vi "Autonomous Independent V.3.0.vi"() -> ()   [LabVIEW 2017]
doc: "This VI is called when autonomous begins, and will automatically be terminated when autonomous ends. You can carry out timed or sensor driven robot movement independently without needing to return to the caller."
uses:
  <vilib>/Rock Robotics/Network Tables/NT Read String.vi
  Robot Global Data V.3.0.vi
panel:
  out "Collector and Drive Loop Run Speed":dbl
  # "Be sure to right-click and choose Data Operations>>Make Current Value default if you want to save the array values with the VI"
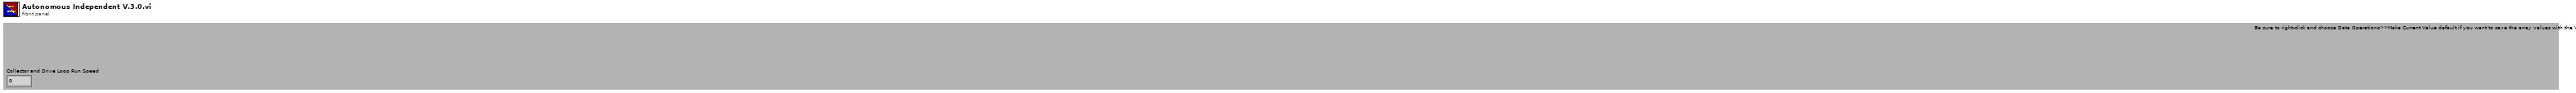
[diagram p1: front panel]
types:
  T1 = typedef "WPI_GyroDevRef.ctl" = cluster{"DevStatus":errorcluster, "Analog Channel":T2, "Gain (VoltsPerDegree/Second)":dbl, "Gyro Type":enum16{"Analog", "XRS450"}, "Handle":i32, "SPI Bus":T3, "Device Found":bool, "Sample Rate":dbl, "Calibrate On Open":bool, "Offset":dbl}
  T2 = typedef "FPGA_AIChannel.ctl" = enum8{"AI 0", "AI 1", "AI 2", "AI 3", "AI MXP 0", "AI MXP 1", "AI MXP 2", "AI MXP 3", "Invalid"}
  T3 = typedef "spi_bus.ctl" = enum16{"SPI On-Board, CS0", "SPI On-Board, CS1", "SPI On-Board, CS2", "SPI On-Board, CS3", "SPI MXP", "Invalid"}
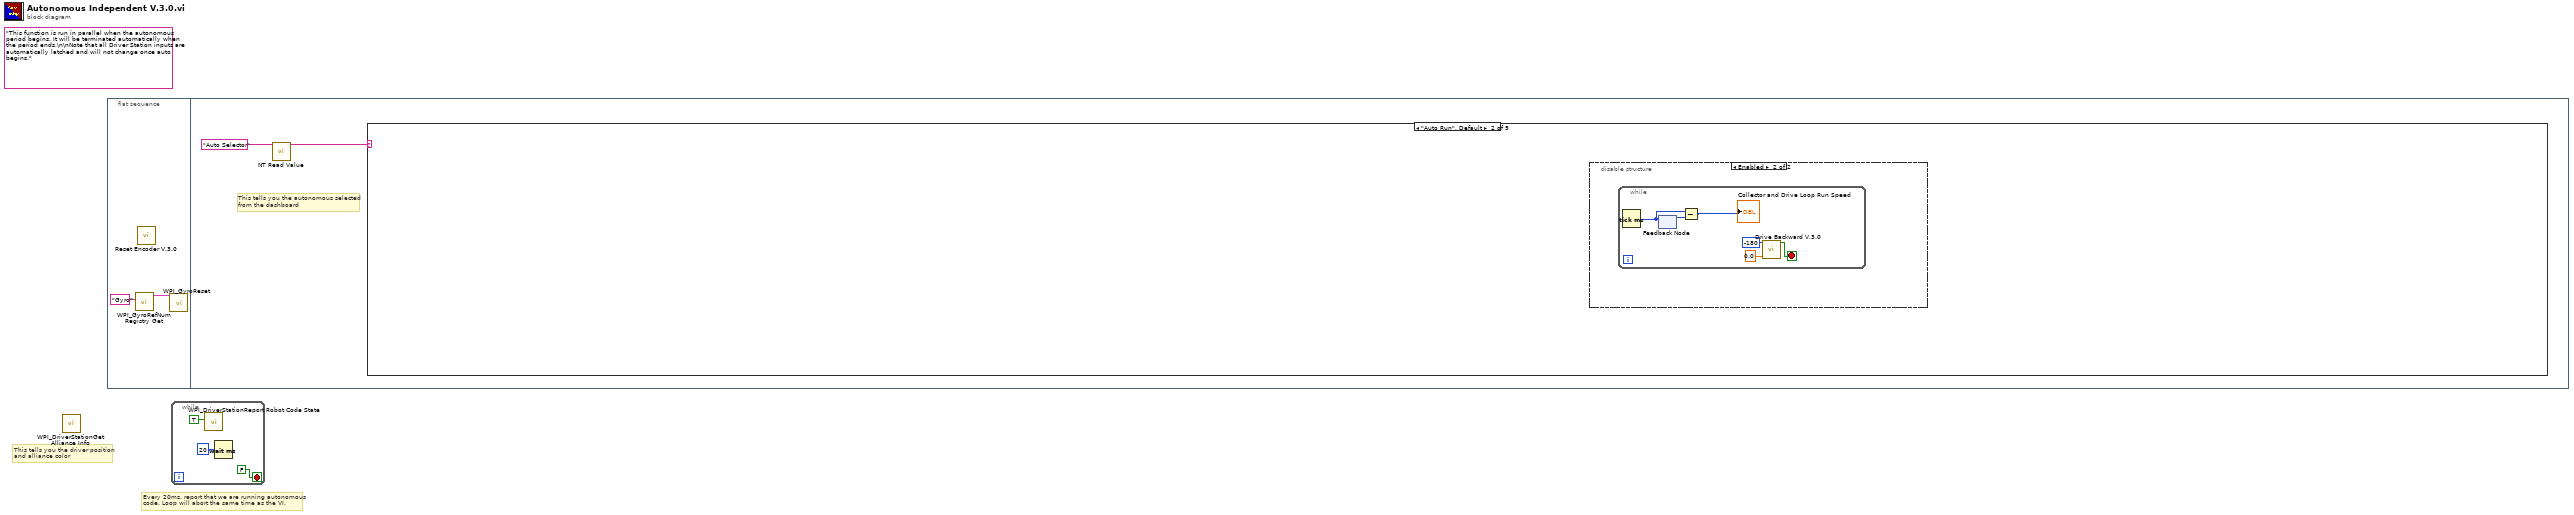
[diagram p0: block diagram]
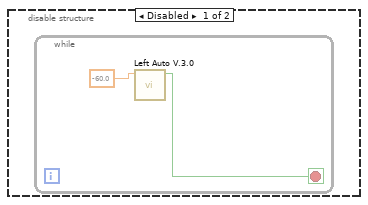
[diagram p3: hidden frame]
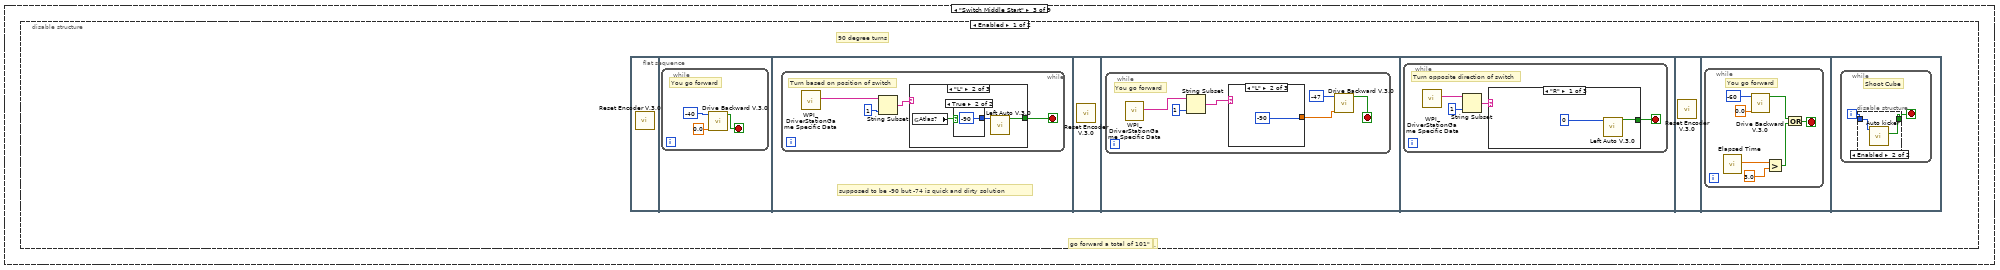
[diagram p4: hidden frame]
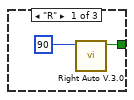
[diagram p5: hidden frame]
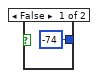
[diagram p6: hidden frame]
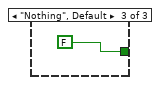
[diagram p7: hidden frame]
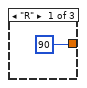
[diagram p8: hidden frame]
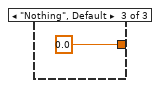
[diagram p9: hidden frame]
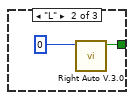
[diagram p10: hidden frame]
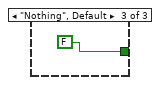
[diagram p11: hidden frame]
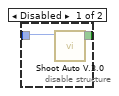
[diagram p12: hidden frame]
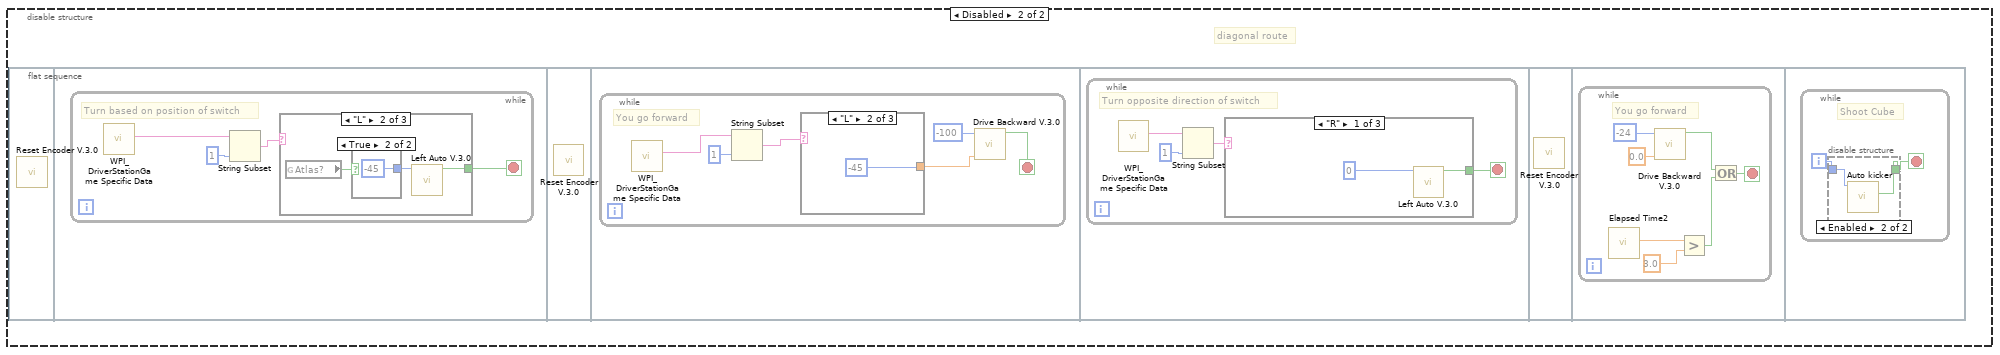
[diagram p13: hidden frame]
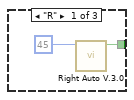
[diagram p14: hidden frame]
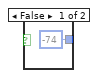
[diagram p15: hidden frame]
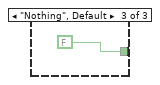
[diagram p16: hidden frame]
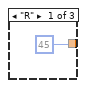
[diagram p17: hidden frame]
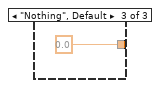
[diagram p18: hidden frame]
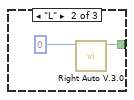
[diagram p19: hidden frame]
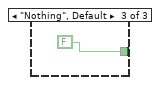
[diagram p20: hidden frame]
diagram:
  (unwired) "This function is run in parallel when the autonomous period begins. It will be terminated automatically when the period ends.\n\nNote that all Driver Station inputs are automatically latched and will not change once auto begins."
  # "This tells you the driver position\nand alliance color"
  # "Every 20ms, report that we are running autonomous\ncode. Loop will abort the same time as the VI."
  n1 = call <vilib>:"WPI_DriverStationGet Alliance Info.vi"() -> ()  [unwired: 12 out]
  n2 = flat-sequence {
    frame #0 {
      n3 = call <vilib>:"WPI_GyroRefNum Registry Get.vi"("refnum name"="Gyro") -> ("GyroDevRef"=w2:T1)  [unwired: 9 in, 1 out]
      n4 = call "Reset Encoder V.3.0.vi"() -> ()  [unwired: 12 in]
      n5 = call <vilib>:"WPI_GyroReset.vi"("GyroDevRef"=w2) -> ()  [unwired: 9 in, 2 out]
    }
    frame #1 {
      # "This tells you the autonomous selected\nfrom the dashboard"
      n6 = call-poly <vilib>:"NT Read Value.vi"("Name"="Auto Selector") -> ("String"=w3:string)  [unwired: 9 in, 1 out]
      n7 = case shown="\"Auto Run\", Default" w3 {
        frame "Nothing" {
          # "You can put your main auto here, or you can right-click on the case and make any\nother frame be the default case."
          # "This is the frame that will execute if no selection is made, or if it is not recognized"
        }
        frame "Auto Run", Default {
          n8 = disable-structure shown="Enabled" {
            frame Disabled {
              n9 = while {
                stop <- w5 stop-if-true
                n10 = call "Left Auto V.3.0.vi"("Desired Angle"=-60.0) -> ("Stop"=w5:bool)  [unwired: 10 in]
              }
            }
            frame Enabled {
              n11 = while {
                stop <- w11 stop-if-true
                n12 = Tick Count (ms)() -> (millisecond timer value=w9:u32)
                n13 = feedback #1() -> (w10:u32)  [unwired: 1 in]
                n14 = feedback-in #1(w9) -> ()
                n15 = Subtract(x=w9, y=w10) -> (x-y=→"Collector and Drive Loop Run Speed":u32)
                n16 = call "Drive Backward V.3.0.vi"("Desired Angle"=0.0, "Encoder Distance (in.)"=-180) -> ("Stop"=w11:bool)  [unwired: 9 in]
              }
            }
          }
        }
        frame "Switch Middle Start" {
          n17 = disable-structure shown="Enabled" {
            frame Enabled {
              # "90 degree turns"
              # "."
              # "go forward a total of 101\""
              n18 = flat-sequence {
                frame #0 {
                  n19 = call "Reset Encoder V.3.0.vi"() -> ()  [unwired: 12 in]
                }
                frame #1 {
                  n20 = while {
                    stop <- w14 stop-if-true
                    # "You go forward"
                    n21 = call "Drive Backward V.3.0.vi"("Desired Angle"=0.0, "Encoder Distance (in.)"=-40) -> ("Stop"=w14:bool)  [unwired: 9 in]
                  }
                }
                frame #2 {
                  # "supposed to be -90 but -74 is quick and dirty solution"
                  n22 = while {
                    stop <- w16 stop-if-true
                    # "Turn based on position of switch"
                    n23 = call <vilib>:"WPI_DriverStationGame Specific Data.vi"() -> ("Game Specific Data"=w19:string)  [unwired: 11 in]
                    n24 = String Subset(string=w19, length (rest)=1 ("length (rest)")) -> (substring=w17:string)  [unwired: 1 in]
                    n25 = case shown="\"L\"" w17 {
                      tunnel: [w20 w23 FALSE] -> w16
                      frame "R" {
                        n26 = call "Right Auto V.3.0.vi"("Desired Angle"=90) -> ("Stop"=w20:bool)  [unwired: 9 in]
                      }
                      frame "L" {
                        n27 = global read "Robot Global Data V.3.0.vi" "Atlas?"() -> (w22:bool)
                        n28 = case shown="True" w22 {
                          tunnel: [-74 -90] -> w24
                          frame False {
                          }
                          frame True {
                          }
                        }
                        n29 = call "Left Auto V.3.0.vi"("Desired Angle"=w24) -> ("Stop"=w23:bool)  [unwired: 10 in]
                      }
                      frame "Nothing", Default {
                      }
                    }
                  }
                }
                frame #3 {
                  n30 = call "Reset Encoder V.3.0.vi"() -> ()  [unwired: 12 in]
                }
                frame #4 {
                  n31 = while {
                    stop <- w32 stop-if-true
                    # "You go forward"
                    n32 = call <vilib>:"WPI_DriverStationGame Specific Data.vi"() -> ("Game Specific Data"=w30:string)  [unwired: 11 in]
                    n33 = String Subset(string=w30, length (rest)=1 ("length (rest)")) -> (substring=w31:string)  [unwired: 1 in]
                    n34 = case shown="\"L\"" w31 {
                      tunnel: [90 -90 0.0] -> w28
                      frame "R" {
                      }
                      frame "L" {
                      }
                      frame "Nothing", Default {
                      }
                    }
                    n35 = call "Drive Backward V.3.0.vi"("Desired Angle"=w28, "Encoder Distance (in.)"=-47) -> ("Stop"=w32:bool)  [unwired: 9 in]
                  }
                }
                frame #5 {
                  n36 = while {
                    stop <- w37 stop-if-true
                    # "Turn opposite direction of switch"
                    n37 = call <vilib>:"WPI_DriverStationGame Specific Data.vi"() -> ("Game Specific Data"=w40:string)  [unwired: 11 in]
                    n38 = String Subset(string=w40, length (rest)=1 ("length (rest)")) -> (substring=w38:string)  [unwired: 1 in]
                    n39 = case shown="\"R\"" w38 {
                      tunnel: [w41 w43 FALSE] -> w37
                      frame "R" {
                        n40 = call "Left Auto V.3.0.vi"("Desired Angle"=0) -> ("Stop"=w41:bool)  [unwired: 10 in]
                      }
                      frame "L" {
                        n41 = call "Right Auto V.3.0.vi"("Desired Angle"=0) -> ("Stop"=w43:bool)  [unwired: 9 in]
                      }
                      frame "Nothing", Default {
                      }
                    }
                  }
                }
                frame #6 {
                  n42 = call "Reset Encoder V.3.0.vi"() -> ()  [unwired: 12 in]
                }
                frame #7 {
                  n43 = while {
                    stop <- w50 stop-if-true
                    # "You go forward"
                    n44 = call "Elapsed Time"() -> ("Elapsed Time (s)"=w48:dbl)  [unwired: 12 in, 7 out]
                    n45 = call "Drive Backward V.3.0.vi"("Desired Angle"=0.0, "Encoder Distance (in.)"=-60) -> ("Stop"=w46:bool)  [unwired: 9 in]
                    n46 = Greater?(x=w48, y=3.0) -> (0:w47:bool)
                    n47 = Or(x=w46, y=w47) -> (x .or. y?=w50:bool)
                  }
                }
                frame #8 {
                  n48 = while {
                    i -> [w54]
                    stop <- w53 stop-if-true
                    # "Shoot Cube"
                    n49 = disable-structure shown="Enabled" {
                      disable-tunnel: w54 -> [w56 w58]
                      disable-tunnel: [w55 w57] -> w53
                      frame Disabled {
                        n50 = call "Shoot Auto V.3.0.vi"("Iteration"=w56) -> ("Stop"=w55:bool)  [unwired: 10 in]
                      }
                      frame Enabled {
                        n51 = call "Auto kicker.vi"("Iteration"=w58) -> ("Stop"=w57:bool)  [unwired: 10 in]
                      }
                    }
                  }
                }
              }
            }
            frame Disabled {
              # "diagonal route"
              n52 = flat-sequence {
                frame #0 {
                  n53 = call "Reset Encoder V.3.0.vi"() -> ()  [unwired: 12 in]
                }
                frame #1 {
                  n54 = while {
                    stop <- w59 stop-if-true
                    # "Turn based on position of switch"
                    n55 = call <vilib>:"WPI_DriverStationGame Specific Data.vi"() -> ("Game Specific Data"=w62:string)  [unwired: 11 in]
                    n56 = String Subset(string=w62, length (rest)=1 ("length (rest)")) -> (substring=w60:string)  [unwired: 1 in]
                    n57 = case shown="\"L\"" w60 {
                      tunnel: [w63 w66 FALSE] -> w59
                      frame "R" {
                        n58 = call "Right Auto V.3.0.vi"("Desired Angle"=45) -> ("Stop"=w63:bool)  [unwired: 9 in]
                      }
                      frame "L" {
                        n59 = global read "Robot Global Data V.3.0.vi" "Atlas?"() -> (w65:bool)
                        n60 = case shown="True" w65 {
                          tunnel: [-74 -45] -> w67
                          frame False {
                          }
                          frame True {
                          }
                        }
                        n61 = call "Left Auto V.3.0.vi"("Desired Angle"=w67) -> ("Stop"=w66:bool)  [unwired: 10 in]
                      }
                      frame "Nothing", Default {
                      }
                    }
                  }
                }
                frame #2 {
                  n62 = call "Reset Encoder V.3.0.vi"() -> ()  [unwired: 12 in]
                }
                frame #3 {
                  n63 = while {
                    stop <- w75 stop-if-true
                    # "You go forward"
                    n64 = call <vilib>:"WPI_DriverStationGame Specific Data.vi"() -> ("Game Specific Data"=w73:string)  [unwired: 11 in]
                    n65 = String Subset(string=w73, length (rest)=1 ("length (rest)")) -> (substring=w74:string)  [unwired: 1 in]
                    n66 = case shown="\"L\"" w74 {
                      tunnel: [45 -45 0.0] -> w71
                      frame "R" {
                      }
                      frame "L" {
                      }
                      frame "Nothing", Default {
                      }
                    }
                    n67 = call "Drive Backward V.3.0.vi"("Desired Angle"=w71, "Encoder Distance (in.)"=-100) -> ("Stop"=w75:bool)  [unwired: 9 in]
                  }
                }
                frame #4 {
                  n68 = while {
                    stop <- w80 stop-if-true
                    # "Turn opposite direction of switch"
                    n69 = call <vilib>:"WPI_DriverStationGame Specific Data.vi"() -> ("Game Specific Data"=w83:string)  [unwired: 11 in]
                    n70 = String Subset(string=w83, length (rest)=1 ("length (rest)")) -> (substring=w81:string)  [unwired: 1 in]
                    n71 = case shown="\"R\"" w81 {
                      tunnel: [w84 w86 FALSE] -> w80
                      frame "R" {
                        n72 = call "Left Auto V.3.0.vi"("Desired Angle"=0) -> ("Stop"=w84:bool)  [unwired: 10 in]
                      }
                      frame "L" {
                        n73 = call "Right Auto V.3.0.vi"("Desired Angle"=0) -> ("Stop"=w86:bool)  [unwired: 9 in]
                      }
                      frame "Nothing", Default {
                      }
                    }
                  }
                }
                frame #5 {
                  n74 = call "Reset Encoder V.3.0.vi"() -> ()  [unwired: 12 in]
                }
                frame #6 {
                  n75 = while {
                    stop <- w93 stop-if-true
                    # "You go forward"
                    n76 = call "Elapsed Time2"() -> ("Elapsed Time (s)"=w91:dbl)  [unwired: 12 in, 7 out]
                    n77 = call "Drive Backward V.3.0.vi"("Desired Angle"=0.0, "Encoder Distance (in.)"=-24) -> ("Stop"=w89:bool)  [unwired: 9 in]
                    n78 = Greater?(x=w91, y=3.0) -> (0:w90:bool)
                    n79 = Or(x=w89, y=w90) -> (x .or. y?=w93:bool)
                  }
                }
                frame #7 {
                  n80 = while {
                    i -> [w97]
                    stop <- w96 stop-if-true
                    # "Shoot Cube"
                    n81 = disable-structure shown="Enabled" {
                      disable-tunnel: w97 -> [w99 w101]
                      disable-tunnel: [w98 w100] -> w96
                      frame Disabled {
                        n82 = call "Shoot Auto V.3.0.vi"("Iteration"=w99) -> ("Stop"=w98:bool)  [unwired: 10 in]
                      }
                      frame Enabled {
                        n83 = call "Auto kicker.vi"("Iteration"=w101) -> ("Stop"=w100:bool)  [unwired: 10 in]
                      }
                    }
                  }
                }
              }
            }
          }
        }
        frame "Switch Optimize Left Start" {
          # "Read Switch Side"
          n84 = call <vilib>:"WPI_DriverStationGame Specific Data.vi"() -> ("Game Specific Data"=w104:string)  [unwired: 11 in]
          n85 = String Subset(string=w104, length (rest)=1 ("length (rest)")) -> (substring=w102:string)  [unwired: 1 in]
          n86 = case shown="\"R\"" w102 {
            frame "Nothing", Default {
            }
            frame "R" {
              w106 = 1 ("length (rest)")
              # "switch on other side, check scale"
              n87 = call <vilib>:"WPI_DriverStationGame Specific Data.vi"() -> ("Game Specific Data"=w107:string)  [unwired: 11 in]
              n88 = String Subset(string=w107, offset (0)=w106, length (rest)=w106) -> (substring=w105:string)
              n89 = case shown="\"L\"" w105 {
                frame "Nothing", Default {
                }
                frame "L" {
                  # "Scale on our side, do it"
                  n90 = flat-sequence {
                    frame #0 {
                      n91 = call "Reset Encoder V.3.0.vi"() -> ()  [unwired: 12 in]
                    }
                    frame #1 {
                      n92 = while {
                        stop <- w109 stop-if-true
                        # "You go forward"
                        n93 = call "Drive Backward V.3.0.vi"("Desired Angle"=0.0, "Encoder Distance (in.)"=-262) -> ("Stop"=w109:bool)  [unwired: 9 in]
                      }
                    }
                    frame #2 {
                      n94 = flat-sequence {
                        frame #0 {
                          n95 = while {
                            stop <- w113 stop-if-true
                            # "Turn right slightly"
                            n96 = call "Right Auto V.3.0.vi"("Desired Angle"=60) -> ("Stop"=w113:bool)  [unwired: 9 in]
                          }
                        }
                        frame #1 {
                          n97 = call "Reset Encoder V.3.0.vi"() -> ()  [unwired: 12 in]
                        }
                        frame #2 {
                          n98 = while {
                            stop <- w116 stop-if-true
                            # "Forward"
                            n99 = call "Drive Backward V.3.0.vi"("Desired Angle"=60.0, "Encoder Distance (in.)"=-16) -> ("Stop"=w116:bool)  [unwired: 9 in]
                          }
                        }
                      }
                      n100 = while {
                        stop <- w111 stop-if-true
                        # "Raise Darts"
                        n101 = call "Dart Auto V.3.0.vi"() -> ("Stop"=w111:bool)  [unwired: 11 in]
                      }
                    }
                    frame #3 {
                      n102 = call "Reset Encoder V.3.0.vi"() -> ()  [unwired: 12 in]
                    }
                    frame #4 {
                      n103 = disable-structure shown="Enabled" {
                        frame Enabled {
                          n104 = while {
                            stop <- w121 stop-if-true
                            # "Move Backward"
                            n105 = call "Forward Auto V.3.0.vi"("Desired Angle"=90.0, "Encoder Distance (in.)"=30.0 ("Encoder Distance")) -> ("Stop"=w121:bool)  [unwired: 9 in]
                          }
                          n106 = flat-sequence {
                            frame #0 {
                              n107 = while {
                                i -> [w118]
                                stop <- w117 stop-if-true
                                # "Shoot Cube"
                                n108 = call "Shoot Auto V.3.0.vi"("Iteration"=w118) -> ("Stop"=w117:bool)  [unwired: 10 in]
                              }
                            }
                            frame #1 {
                              n109 = while {
                                stop <- w119 stop-if-true
                                n110 = call "Auto Arms Down V.3.0.vi"() -> ("Stop"=w119:bool)  [unwired: 11 in]
                              }
                            }
                          }
                        }
                        frame Disabled {
                        }
                      }
                    }
                    frame #5 {
                      n111 = disable-structure shown="Disabled" {
                        frame Disabled {
                          n112 = while {
                            stop <- w124 stop-if-true
                            # "Turn right slightly"
                            n113 = call "Right Auto V.3.0.vi"("Desired Angle"=-30) -> ("Stop"=w124:bool)  [unwired: 9 in]
                          }
                        }
                        frame Enabled {
                        }
                      }
                    }
                  }
                }
                frame "R" {
                  # "Scale on other side, do it anyway"
                  n114 = flat-sequence {
                    frame #0 {
                      n115 = call "Reset Encoder V.3.0.vi"() -> ()  [unwired: 12 in]
                    }
                    frame #1 {
                      n116 = while {
                        stop <- w126 stop-if-true
                        # "Forward"
                        n117 = call "Drive Backward V.3.0.vi"("Desired Angle"=0.0, "Encoder Distance (in.)"=-232) -> ("Stop"=w126:bool)  [unwired: 9 in]
                      }
                    }
                    frame #2 {
                      n118 = while {
                        stop <- w129 stop-if-true
                        # "Right"
                        n119 = call "Right Auto V.3.0.vi"("Desired Angle"=90) -> ("Stop"=w129:bool)  [unwired: 9 in]
                      }
                    }
                    frame #3 {
                      n120 = call "Reset Encoder V.3.0.vi"() -> ()  [unwired: 12 in]
                    }
                    frame #4 {
                      n121 = while {
                        stop <- w131 stop-if-true
                        # "Forward"
                        n122 = call "Drive Backward V.3.0.vi"("Desired Angle"=90.0, "Encoder Distance (in.)"=-200) -> ("Stop"=w131:bool)  [unwired: 9 in]
                      }
                    }
                    frame #5 {
                      n123 = flat-sequence {
                        frame #0 {
                          n124 = while {
                            stop <- w135 stop-if-true
                            # "Left"
                            n125 = call "Left Auto V.3.0.vi"("Desired Angle"=0) -> ("Stop"=w135:bool)  [unwired: 10 in]
                          }
                        }
                        frame #1 {
                          n126 = call "Reset Encoder V.3.0.vi"() -> ()  [unwired: 12 in]
                        }
                        frame #2 {
                          n127 = disable-structure shown="Disabled" {
                            frame Disabled {
                              n128 = while {
                                stop <- w138 stop-if-true
                                # "Forward"
                                n129 = call "Drive Backward V.3.0.vi"("Desired Angle"=0.0, "Encoder Distance (in.)"=-49) -> ("Stop"=w138:bool)  [unwired: 9 in]
                              }
                            }
                            frame Enabled {
                            }
                          }
                        }
                      }
                      n130 = while {
                        stop <- w133 stop-if-true
                        # "Raise Darts"
                        n131 = call "Dart Auto V.3.0.vi"() -> ("Stop"=w133:bool)  [unwired: 11 in]
                      }
                    }
                    frame #6 {
                      n132 = disable-structure shown="Disabled" {
                        frame Disabled {
                          n133 = while {
                            i -> [w140]
                            stop <- w139 stop-if-true
                            # "Shoot Cube"
                            n134 = call "Shoot Auto V.3.0.vi"("Iteration"=w140) -> ("Stop"=w139:bool)  [unwired: 10 in]
                          }
                        }
                        frame Enabled {
                        }
                      }
                    }
                    frame #7 {
                      n135 = call "Reset Encoder V.3.0.vi"() -> ()  [unwired: 12 in]
                    }
                    frame #8 {
                      n136 = disable-structure shown="Disabled" {
                        frame Disabled {
                          n137 = while {
                            stop <- w143 stop-if-true
                            # "Move Backward"
                            n138 = call "Forward Auto V.3.0.vi"("Desired Angle"=0.0, "Encoder Distance (in.)"=10.0 ("Encoder Distance")) -> ("Stop"=w143:bool)  [unwired: 9 in]
                          }
                          n139 = while {
                            stop <- w141 stop-if-true
                            n140 = call "Auto Arms Down V.3.0.vi"() -> ("Stop"=w141:bool)  [unwired: 11 in]
                          }
                        }
                        frame Enabled {
                        }
                      }
                    }
                  }
                }
              }
            }
            frame "L" {
              # "Switch on our side, do switch"
              n141 = flat-sequence {
                frame #0 {
                  n142 = call "Reset Encoder V.3.0.vi"() -> ()  [unwired: 12 in]
                }
                frame #1 {
                  n143 = while {
                    stop <- w147 stop-if-true
                    # "was -183"
                    n144 = call "Drive Backward V.3.0.vi"("Desired Angle"=0.0, "Encoder Distance (in.)"=-162.0) -> ("Stop"=w147:bool)  [unwired: 9 in]
                  }
                }
                frame #2 {
                  n145 = while {
                    stop <- w149 stop-if-true
                    n146 = call "Right Auto V.3.0.vi"("Desired Angle"=90.0) -> ("Stop"=w149:bool)  [unwired: 9 in]
                  }
                }
                frame #3 {
                  n147 = call "Reset Encoder V.3.0.vi"() -> ()  [unwired: 12 in]
                }
                frame #4 {
                  n148 = while {
                    stop <- w150 stop-if-true
                    # "was  -16"
                    n149 = call "Drive Backward V.3.0.vi"("Desired Angle"=90.0, "Encoder Distance (in.)"=-22.0) -> ("Stop"=w150:bool)  [unwired: 9 in]
                  }
                }
                frame #5 {
                  n150 = while {
                    i -> [w153]
                    stop <- w154 stop-if-true
                    n151 = call "Shoot Auto V.3.0.vi"("Iteration"=w153) -> ("Stop"=w154:bool)  [unwired: 10 in]
                  }
                }
              }
            }
          }
        }
        frame "Switch Optimize Right Start" {
          # "Read Switch"
          n152 = call <vilib>:"WPI_DriverStationGame Specific Data.vi"() -> ("Game Specific Data"=w157:string)  [unwired: 11 in]
          n153 = String Subset(string=w157, length (rest)=1 ("length (rest)")) -> (substring=w155:string)  [unwired: 1 in]
          n154 = case shown="\"L\"" w155 {
            frame "Nothing", Default {
            }
            frame "R" {
              # "Switch on our side, do it"
              n155 = flat-sequence {
                frame #0 {
                  n156 = call "Reset Encoder V.3.0.vi"() -> ()  [unwired: 12 in]
                }
                frame #1 {
                  n157 = while {
                    stop <- w160 stop-if-true
                    # "was -183"
                    n158 = call "Drive Backward V.3.0.vi"("Desired Angle"=0.0, "Encoder Distance (in.)"=-162.0) -> ("Stop"=w160:bool)  [unwired: 9 in]
                  }
                }
                frame #2 {
                  n159 = while {
                    stop <- w162 stop-if-true
                    n160 = call "Right Auto V.3.0.vi"("Desired Angle"=90.0) -> ("Stop"=w162:bool)  [unwired: 9 in]
                  }
                }
                frame #3 {
                  n161 = call "Reset Encoder V.3.0.vi"() -> ()  [unwired: 12 in]
                }
                frame #4 {
                  n162 = while {
                    stop <- w163 stop-if-true
                    # "was  -16"
                    n163 = call "Drive Backward V.3.0.vi"("Desired Angle"=90.0, "Encoder Distance (in.)"=-22.0) -> ("Stop"=w163:bool)  [unwired: 9 in]
                  }
                }
                frame #5 {
                  n164 = while {
                    i -> [w166]
                    stop <- w167 stop-if-true
                    n165 = call "Shoot Auto V.3.0.vi"("Iteration"=w166) -> ("Stop"=w167:bool)  [unwired: 10 in]
                  }
                }
              }
            }
            frame "L" {
              w169 = 1 ("length (rest)")
              # "Switch on wrong side, read\nscale"
              n166 = call <vilib>:"WPI_DriverStationGame Specific Data.vi"() -> ("Game Specific Data"=w170:string)  [unwired: 11 in]
              n167 = String Subset(string=w170, offset (0)=w169, length (rest)=w169) -> (substring=w168:string)
              n168 = case shown="\"R\"" w168 {
                frame "Nothing", Default {
                }
                frame "R" {
                  # "Scale on same side - do it"
                  n169 = flat-sequence {
                    frame #0 {
                      n170 = call "Reset Encoder V.3.0.vi"() -> ()  [unwired: 12 in]
                    }
                    frame #1 {
                      # "was -277"
                      n171 = while {
                        stop <- w172 stop-if-true
                        # "You go forward"
                        n172 = call "Drive Backward V.3.0.vi"("Desired Angle"=0.0, "Encoder Distance (in.)"=-262) -> ("Stop"=w172:bool)  [unwired: 9 in]
                      }
                    }
                    frame #2 {
                      n173 = flat-sequence {
                        frame #0 {
                          n174 = while {
                            stop <- w176 stop-if-true
                            # "Turn LEFT"
                            n175 = call "Left Auto V.3.0.vi"("Desired Angle"=-60) -> ("Stop"=w176:bool)  [unwired: 10 in]
                          }
                        }
                        frame #1 {
                          n176 = call "Reset Encoder V.3.0.vi"() -> ()  [unwired: 12 in]
                        }
                        frame #2 {
                          n177 = while {
                            stop <- w179 stop-if-true
                            # "Forward"
                            n178 = call "Drive Backward V.3.0.vi"("Desired Angle"=-60.0, "Encoder Distance (in.)"=-16) -> ("Stop"=w179:bool)  [unwired: 9 in]
                          }
                        }
                      }
                      n179 = while {
                        stop <- w174 stop-if-true
                        # "Raise Darts"
                        n180 = call "Dart Auto V.3.0.vi"() -> ("Stop"=w174:bool)  [unwired: 11 in]
                      }
                    }
                    frame #3 {
                      n181 = call "Reset Encoder V.3.0.vi"() -> ()  [unwired: 12 in]
                    }
                    frame #4 {
                      n182 = disable-structure shown="Enabled" {
                        frame Enabled {
                          n183 = while {
                            stop <- w184 stop-if-true
                            # "Move Backward"
                            n184 = call "Forward Auto V.3.0.vi"("Desired Angle"=90.0, "Encoder Distance (in.)"=30.0 ("Encoder Distance")) -> ("Stop"=w184:bool)  [unwired: 9 in]
                          }
                          n185 = flat-sequence {
                            frame #0 {
                              n186 = while {
                                i -> [w181]
                                stop <- w180 stop-if-true
                                # "Shoot Cube"
                                n187 = call "Shoot Auto V.3.0.vi"("Iteration"=w181) -> ("Stop"=w180:bool)  [unwired: 10 in]
                              }
                            }
                            frame #1 {
                              n188 = while {
                                stop <- w182 stop-if-true
                                n189 = call "Auto Arms Down V.3.0.vi"() -> ("Stop"=w182:bool)  [unwired: 11 in]
                              }
                            }
                          }
                        }
                        frame Disabled {
                        }
                      }
                    }
                    frame #5 {
                      n190 = disable-structure shown="Disabled" {
                        frame Disabled {
                          n191 = while {
                            stop <- w187 stop-if-true
                            # "Turn right slightly"
                            n192 = call "Right Auto V.3.0.vi"("Desired Angle"=-30) -> ("Stop"=w187:bool)  [unwired: 9 in]
                          }
                        }
                        frame Enabled {
                        }
                      }
                    }
                  }
                }
                frame "L" {
                  # "Scale on wrong side, do it anyway"
                  n193 = flat-sequence {
                    frame #0 {
                      n194 = call "Reset Encoder V.3.0.vi"() -> ()  [unwired: 12 in]
                    }
                    frame #1 {
                      n195 = while {
                        stop <- w189 stop-if-true
                        # "Forward"
                        n196 = call "Drive Backward V.3.0.vi"("Desired Angle"=0.0, "Encoder Distance (in.)"=-232) -> ("Stop"=w189:bool)  [unwired: 9 in]
                      }
                    }
                    frame #2 {
                      n197 = while {
                        stop <- w192 stop-if-true
                        # "Right"
                        n198 = call "Left Auto V.3.0.vi"("Desired Angle"=-90) -> ("Stop"=w192:bool)  [unwired: 10 in]
                      }
                    }
                    frame #3 {
                      n199 = call "Reset Encoder V.3.0.vi"() -> ()  [unwired: 12 in]
                    }
                    frame #4 {
                      n200 = while {
                        stop <- w194 stop-if-true
                        # "Forward"
                        n201 = call "Drive Backward V.3.0.vi"("Desired Angle"=-90.0, "Encoder Distance (in.)"=-200) -> ("Stop"=w194:bool)  [unwired: 9 in]
                      }
                    }
                    frame #5 {
                      n202 = flat-sequence {
                        frame #0 {
                          n203 = while {
                            stop <- w198 stop-if-true
                            # "Left"
                            n204 = call "Right Auto V.3.0.vi"("Desired Angle"=0) -> ("Stop"=w198:bool)  [unwired: 9 in]
                          }
                        }
                        frame #1 {
                          n205 = call "Reset Encoder V.3.0.vi"() -> ()  [unwired: 12 in]
                        }
                        frame #2 {
                          n206 = disable-structure shown="Disabled" {
                            frame Disabled {
                              n207 = while {
                                stop <- w201 stop-if-true
                                # "Forward"
                                n208 = call "Drive Backward V.3.0.vi"("Desired Angle"=0.0, "Encoder Distance (in.)"=-49) -> ("Stop"=w201:bool)  [unwired: 9 in]
                              }
                            }
                            frame Enabled {
                            }
                          }
                        }
                      }
                      n209 = while {
                        stop <- w196 stop-if-true
                        # "Raise Darts"
                        n210 = call "Dart Auto V.3.0.vi"() -> ("Stop"=w196:bool)  [unwired: 11 in]
                      }
                    }
                    frame #6 {
                      n211 = disable-structure shown="Disabled" {
                        frame Disabled {
                          n212 = while {
                            i -> [w203]
                            stop <- w202 stop-if-true
                            # "Shoot Cube"
                            n213 = call "Shoot Auto V.3.0.vi"("Iteration"=w203) -> ("Stop"=w202:bool)  [unwired: 10 in]
                          }
                        }
                        frame Enabled {
                        }
                      }
                    }
                    frame #7 {
                      n214 = call "Reset Encoder V.3.0.vi"() -> ()  [unwired: 12 in]
                    }
                    frame #8 {
                      n215 = disable-structure shown="Disabled" {
                        frame Disabled {
                          n216 = while {
                            stop <- w206 stop-if-true
                            # "Move Backward"
                            n217 = call "Forward Auto V.3.0.vi"("Desired Angle"=0.0, "Encoder Distance (in.)"=10.0 ("Encoder Distance")) -> ("Stop"=w206:bool)  [unwired: 9 in]
                          }
                          n218 = while {
                            stop <- w204 stop-if-true
                            n219 = call "Auto Arms Down V.3.0.vi"() -> ("Stop"=w204:bool)  [unwired: 11 in]
                          }
                        }
                        frame Enabled {
                        }
                      }
                    }
                  }
                }
              }
            }
          }
        }
        frame "Left Start Always Scale" {
          w208 = 1 ("length (rest)")
          n220 = call <vilib>:"WPI_DriverStationGame Specific Data.vi"() -> ("Game Specific Data"=w210:string)  [unwired: 11 in]
          n221 = String Subset(string=w210, offset (0)=w208, length (rest)=w208) -> (substring=w209:string)
          n222 = case shown="\"L\"" w209 {
            frame "R" {
              n223 = disable-structure shown="Enabled" {
                frame Enabled {
                  n224 = flat-sequence {
                    frame #0 {
                      n225 = call "Reset Encoder V.3.0.vi"() -> ()  [unwired: 12 in]
                    }
                    frame #1 {
                      n226 = while {
                        stop <- w212 stop-if-true
                        # "Forward"
                        n227 = call "Drive Backward V.3.0.vi"("Desired Angle"=0.0, "Encoder Distance (in.)"=-232) -> ("Stop"=w212:bool)  [unwired: 9 in]
                      }
                    }
                    frame #2 {
                      n228 = while {
                        stop <- w215 stop-if-true
                        # "Right"
                        n229 = call "Right Auto V.3.0.vi"("Desired Angle"=90) -> ("Stop"=w215:bool)  [unwired: 9 in]
                      }
                    }
                    frame #3 {
                      n230 = call "Reset Encoder V.3.0.vi"() -> ()  [unwired: 12 in]
                    }
                    frame #4 {
                      n231 = while {
                        stop <- w217 stop-if-true
                        # "Forward"
                        n232 = call "Drive Backward V.3.0.vi"("Desired Angle"=90.0, "Encoder Distance (in.)"=-200) -> ("Stop"=w217:bool)  [unwired: 9 in]
                      }
                    }
                    frame #5 {
                      n233 = flat-sequence {
                        frame #0 {
                          n234 = while {
                            stop <- w221 stop-if-true
                            # "Left"
                            n235 = call "Left Auto V.3.0.vi"("Desired Angle"=0) -> ("Stop"=w221:bool)  [unwired: 10 in]
                          }
                        }
                        frame #1 {
                          n236 = call "Reset Encoder V.3.0.vi"() -> ()  [unwired: 12 in]
                        }
                        frame #2 {
                          n237 = disable-structure shown="Disabled" {
                            frame Disabled {
                              n238 = while {
                                stop <- w224 stop-if-true
                                # "Forward"
                                n239 = call "Drive Backward V.3.0.vi"("Desired Angle"=0.0, "Encoder Distance (in.)"=-49) -> ("Stop"=w224:bool)  [unwired: 9 in]
                              }
                            }
                            frame Enabled {
                            }
                          }
                        }
                      }
                      n240 = while {
                        stop <- w219 stop-if-true
                        # "Raise Darts"
                        n241 = call "Dart Auto V.3.0.vi"() -> ("Stop"=w219:bool)  [unwired: 11 in]
                      }
                    }
                    frame #6 {
                      n242 = disable-structure shown="Disabled" {
                        frame Disabled {
                          n243 = while {
                            i -> [w226]
                            stop <- w225 stop-if-true
                            # "Shoot Cube"
                            n244 = call "Shoot Auto V.3.0.vi"("Iteration"=w226) -> ("Stop"=w225:bool)  [unwired: 10 in]
                          }
                        }
                        frame Enabled {
                        }
                      }
                    }
                    frame #7 {
                      n245 = call "Reset Encoder V.3.0.vi"() -> ()  [unwired: 12 in]
                    }
                    frame #8 {
                      n246 = disable-structure shown="Disabled" {
                        frame Disabled {
                          n247 = while {
                            stop <- w229 stop-if-true
                            # "Move Backward"
                            n248 = call "Forward Auto V.3.0.vi"("Desired Angle"=0.0, "Encoder Distance (in.)"=10.0 ("Encoder Distance")) -> ("Stop"=w229:bool)  [unwired: 9 in]
                          }
                          n249 = while {
                            stop <- w227 stop-if-true
                            n250 = call "Auto Arms Down V.3.0.vi"() -> ("Stop"=w227:bool)  [unwired: 11 in]
                          }
                        }
                        frame Enabled {
                        }
                      }
                    }
                  }
                }
                frame Disabled {
                  n251 = flat-sequence {
                    frame #0 {
                      n252 = call "Reset Encoder V.3.0.vi"() -> ()  [unwired: 12 in]
                    }
                    frame #1 {
                      n253 = while {
                        stop <- w232 stop-if-true
                        # "Forward"
                        n254 = call "Drive Backward V.3.0.vi"("Desired Angle"=0.0, "Encoder Distance (in.)"=-232) -> ("Stop"=w232:bool)  [unwired: 9 in]
                      }
                    }
                    frame #2 {
                      n255 = while {
                        stop <- w235 stop-if-true
                        # "Right"
                        n256 = call "Right Auto V.3.0.vi"("Desired Angle"=90) -> ("Stop"=w235:bool)  [unwired: 9 in]
                      }
                    }
                    frame #3 {
                      n257 = call "Reset Encoder V.3.0.vi"() -> ()  [unwired: 12 in]
                    }
                    frame #4 {
                      n258 = while {
                        stop <- w237 stop-if-true
                        # "Forward"
                        n259 = call "Drive Backward V.3.0.vi"("Desired Angle"=90.0, "Encoder Distance (in.)"=-200) -> ("Stop"=w237:bool)  [unwired: 9 in]
                      }
                    }
                    frame #5 {
                      n260 = flat-sequence {
                        frame #0 {
                          n261 = while {
                            stop <- w241 stop-if-true
                            # "Left"
                            n262 = call "Left Auto V.3.0.vi"("Desired Angle"=0) -> ("Stop"=w241:bool)  [unwired: 10 in]
                          }
                        }
                        frame #1 {
                          n263 = call "Reset Encoder V.3.0.vi"() -> ()  [unwired: 12 in]
                        }
                        frame #2 {
                          n264 = while {
                            stop <- w244 stop-if-true
                            # "Forward"
                            n265 = call "Drive Backward V.3.0.vi"("Desired Angle"=0.0, "Encoder Distance (in.)"=-49) -> ("Stop"=w244:bool)  [unwired: 9 in]
                          }
                        }
                      }
                      n266 = while {
                        stop <- w239 stop-if-true
                        # "Raise Darts"
                        n267 = call "Dart Auto V.3.0.vi"() -> ("Stop"=w239:bool)  [unwired: 11 in]
                      }
                    }
                  }
                }
              }
            }
            frame "L" {
              # "was 277"
              n268 = flat-sequence {
                frame #0 {
                  n269 = call "Reset Encoder V.3.0.vi"() -> ()  [unwired: 12 in]
                }
                frame #1 {
                  n270 = while {
                    stop <- w246 stop-if-true
                    # "You go forward"
                    n271 = call "Drive Backward V.3.0.vi"("Desired Angle"=0.0, "Encoder Distance (in.)"=-262) -> ("Stop"=w246:bool)  [unwired: 9 in]
                  }
                }
                frame #2 {
                  n272 = flat-sequence {
                    frame #0 {
                      n273 = while {
                        stop <- w250 stop-if-true
                        # "Turn right slightly"
                        n274 = call "Right Auto V.3.0.vi"("Desired Angle"=60) -> ("Stop"=w250:bool)  [unwired: 9 in]
                      }
                    }
                    frame #1 {
                      n275 = call "Reset Encoder V.3.0.vi"() -> ()  [unwired: 12 in]
                    }
                    frame #2 {
                      n276 = while {
                        stop <- w253 stop-if-true
                        # "Forward"
                        n277 = call "Drive Backward V.3.0.vi"("Desired Angle"=60.0, "Encoder Distance (in.)"=-16) -> ("Stop"=w253:bool)  [unwired: 9 in]
                      }
                    }
                  }
                  n278 = while {
                    stop <- w248 stop-if-true
                    # "Raise Darts"
                    n279 = call "Dart Auto V.3.0.vi"() -> ("Stop"=w248:bool)  [unwired: 11 in]
                  }
                }
                frame #3 {
                  n280 = call "Reset Encoder V.3.0.vi"() -> ()  [unwired: 12 in]
                }
                frame #4 {
                  n281 = disable-structure shown="Enabled" {
                    frame Enabled {
                      n282 = while {
                        stop <- w258 stop-if-true
                        # "Move Backward"
                        n283 = call "Forward Auto V.3.0.vi"("Desired Angle"=90.0, "Encoder Distance (in.)"=30.0 ("Encoder Distance")) -> ("Stop"=w258:bool)  [unwired: 9 in]
                      }
                      n284 = flat-sequence {
                        frame #0 {
                          n285 = while {
                            i -> [w255]
                            stop <- w254 stop-if-true
                            # "Shoot Cube"
                            n286 = call "Shoot Auto V.3.0.vi"("Iteration"=w255) -> ("Stop"=w254:bool)  [unwired: 10 in]
                          }
                        }
                        frame #1 {
                          n287 = while {
                            stop <- w256 stop-if-true
                            n288 = call "Auto Arms Down V.3.0.vi"() -> ("Stop"=w256:bool)  [unwired: 11 in]
                          }
                        }
                      }
                    }
                    frame Disabled {
                    }
                  }
                }
                frame #5 {
                  n289 = disable-structure shown="Disabled" {
                    frame Disabled {
                      n290 = while {
                        stop <- w261 stop-if-true
                        # "Turn right slightly"
                        n291 = call "Right Auto V.3.0.vi"("Desired Angle"=-30) -> ("Stop"=w261:bool)  [unwired: 9 in]
                      }
                    }
                    frame Enabled {
                    }
                  }
                }
              }
            }
            frame "Nothing", Default {
            }
          }
        }
        frame "Scale Optimize Left Start" {
          w263 = 1 ("length (rest)")
          n292 = call <vilib>:"WPI_DriverStationGame Specific Data.vi"() -> ("Game Specific Data"=w264:string)  [unwired: 11 in]
          n293 = String Subset(string=w264, offset (0)=w263, length (rest)=w263) -> (substring=w262:string)
          n294 = case shown="\"L\"" w262 {
            frame "L" {
              # "same side scale - do scale"
              n295 = flat-sequence {
                frame #0 {
                  n296 = call "Reset Encoder V.3.0.vi"() -> ()  [unwired: 12 in]
                }
                frame #1 {
                  n297 = while {
                    stop <- w266 stop-if-true
                    # "You go forward"
                    n298 = call "Drive Backward V.3.0.vi"("Desired Angle"=0.0, "Encoder Distance (in.)"=-262) -> ("Stop"=w266:bool)  [unwired: 9 in]
                  }
                }
                frame #2 {
                  n299 = flat-sequence {
                    frame #0 {
                      n300 = while {
                        stop <- w270 stop-if-true
                        # "Turn right slightly"
                        n301 = call "Right Auto V.3.0.vi"("Desired Angle"=60) -> ("Stop"=w270:bool)  [unwired: 9 in]
                      }
                    }
                    frame #1 {
                      n302 = call "Reset Encoder V.3.0.vi"() -> ()  [unwired: 12 in]
                    }
                    frame #2 {
                      n303 = while {
                        stop <- w273 stop-if-true
                        # "Forward"
                        n304 = call "Drive Backward V.3.0.vi"("Desired Angle"=60.0, "Encoder Distance (in.)"=-16) -> ("Stop"=w273:bool)  [unwired: 9 in]
                      }
                    }
                  }
                  n305 = while {
                    stop <- w268 stop-if-true
                    # "Raise Darts"
                    n306 = call "Dart Auto V.3.0.vi"() -> ("Stop"=w268:bool)  [unwired: 11 in]
                  }
                }
                frame #3 {
                  n307 = call "Reset Encoder V.3.0.vi"() -> ()  [unwired: 12 in]
                }
                frame #4 {
                  n308 = disable-structure shown="Enabled" {
                    frame Enabled {
                      n309 = while {
                        stop <- w278 stop-if-true
                        # "Move Backward"
                        n310 = call "Forward Auto V.3.0.vi"("Desired Angle"=90.0, "Encoder Distance (in.)"=30.0 ("Encoder Distance")) -> ("Stop"=w278:bool)  [unwired: 9 in]
                      }
                      n311 = flat-sequence {
                        frame #0 {
                          n312 = while {
                            i -> [w275]
                            stop <- w274 stop-if-true
                            # "Shoot Cube"
                            n313 = call "Shoot Auto V.3.0.vi"("Iteration"=w275) -> ("Stop"=w274:bool)  [unwired: 10 in]
                          }
                        }
                        frame #1 {
                          n314 = while {
                            stop <- w276 stop-if-true
                            n315 = call "Auto Arms Down V.3.0.vi"() -> ("Stop"=w276:bool)  [unwired: 11 in]
                          }
                        }
                      }
                    }
                    frame Disabled {
                    }
                  }
                }
                frame #5 {
                  n316 = disable-structure shown="Disabled" {
                    frame Disabled {
                      n317 = while {
                        stop <- w281 stop-if-true
                        # "Turn right slightly"
                        n318 = call "Right Auto V.3.0.vi"("Desired Angle"=-30) -> ("Stop"=w281:bool)  [unwired: 9 in]
                      }
                    }
                    frame Enabled {
                    }
                  }
                }
              }
            }
            frame "R" {
              n319 = call <vilib>:"WPI_DriverStationGame Specific Data.vi"() -> ("Game Specific Data"=w284:string)  [unwired: 11 in]
              n320 = String Subset(string=w284, length (rest)=1 ("length (rest)")) -> (substring=w282:string)  [unwired: 1 in]
              n321 = case shown="\"R\"" w282 {
                frame "Nothing", Default {
                }
                frame "L" {
                  # "opposite side scale same side switch - do switch"
                  n322 = flat-sequence {
                    frame #0 {
                      n323 = call "Reset Encoder V.3.0.vi"() -> ()  [unwired: 12 in]
                    }
                    frame #1 {
                      n324 = while {
                        stop <- w287 stop-if-true
                        n325 = call "Drive Backward V.3.0.vi"("Desired Angle"=0.0, "Encoder Distance (in.)"=-162.0) -> ("Stop"=w287:bool)  [unwired: 9 in]
                      }
                    }
                    frame #2 {
                      n326 = while {
                        stop <- w289 stop-if-true
                        n327 = call "Right Auto V.3.0.vi"("Desired Angle"=90.0) -> ("Stop"=w289:bool)  [unwired: 9 in]
                      }
                    }
                    frame #3 {
                      n328 = call "Reset Encoder V.3.0.vi"() -> ()  [unwired: 12 in]
                    }
                    frame #4 {
                      n329 = while {
                        stop <- w290 stop-if-true
                        n330 = call "Drive Backward V.3.0.vi"("Desired Angle"=90.0, "Encoder Distance (in.)"=-22.0) -> ("Stop"=w290:bool)  [unwired: 9 in]
                      }
                    }
                    frame #5 {
                      n331 = while {
                        i -> [w293]
                        stop <- w294 stop-if-true
                        n332 = call "Shoot Auto V.3.0.vi"("Iteration"=w293) -> ("Stop"=w294:bool)  [unwired: 10 in]
                      }
                    }
                  }
                }
                frame "R" {
                  # "both opposite sides - do scale"
                  n333 = disable-structure shown="Enabled" {
                    frame Enabled {
                      n334 = flat-sequence {
                        frame #0 {
                          n335 = call "Reset Encoder V.3.0.vi"() -> ()  [unwired: 12 in]
                        }
                        frame #1 {
                          n336 = while {
                            stop <- w296 stop-if-true
                            # "Forward"
                            n337 = call "Drive Backward V.3.0.vi"("Desired Angle"=0.0, "Encoder Distance (in.)"=-232) -> ("Stop"=w296:bool)  [unwired: 9 in]
                          }
                        }
                        frame #2 {
                          n338 = while {
                            stop <- w299 stop-if-true
                            # "Right"
                            n339 = call "Right Auto V.3.0.vi"("Desired Angle"=90) -> ("Stop"=w299:bool)  [unwired: 9 in]
                          }
                        }
                        frame #3 {
                          n340 = call "Reset Encoder V.3.0.vi"() -> ()  [unwired: 12 in]
                        }
                        frame #4 {
                          n341 = while {
                            stop <- w301 stop-if-true
                            # "Forward"
                            n342 = call "Drive Backward V.3.0.vi"("Desired Angle"=90.0, "Encoder Distance (in.)"=-200) -> ("Stop"=w301:bool)  [unwired: 9 in]
                          }
                        }
                        frame #5 {
                          n343 = flat-sequence {
                            frame #0 {
                              n344 = while {
                                stop <- w305 stop-if-true
                                # "Left"
                                n345 = call "Left Auto V.3.0.vi"("Desired Angle"=0) -> ("Stop"=w305:bool)  [unwired: 10 in]
                              }
                            }
                            frame #1 {
                              n346 = call "Reset Encoder V.3.0.vi"() -> ()  [unwired: 12 in]
                            }
                            frame #2 {
                              n347 = disable-structure shown="Disabled" {
                                frame Disabled {
                                n348 = while {
                                stop <- w308 stop-if-true
                                # "Forward"
                                n349 = call "Drive Backward V.3.0.vi"("Desired Angle"=0.0, "Encoder Distance (in.)"=-49) -> ("Stop"=w308:bool)  [unwired: 9 in]
                                }
                                }
                                frame Enabled {
                                }
                              }
                            }
                          }
                          n350 = while {
                            stop <- w303 stop-if-true
                            # "Raise Darts"
                            n351 = call "Dart Auto V.3.0.vi"() -> ("Stop"=w303:bool)  [unwired: 11 in]
                          }
                        }
                        frame #6 {
                          n352 = disable-structure shown="Disabled" {
                            frame Disabled {
                              n353 = while {
                                i -> [w310]
                                stop <- w309 stop-if-true
                                # "Shoot Cube"
                                n354 = call "Shoot Auto V.3.0.vi"("Iteration"=w310) -> ("Stop"=w309:bool)  [unwired: 10 in]
                              }
                            }
                            frame Enabled {
                            }
                          }
                        }
                        frame #7 {
                          n355 = call "Reset Encoder V.3.0.vi"() -> ()  [unwired: 12 in]
                        }
                        frame #8 {
                          n356 = disable-structure shown="Disabled" {
                            frame Disabled {
                              n357 = while {
                                stop <- w313 stop-if-true
                                # "Move Backward"
                                n358 = call "Forward Auto V.3.0.vi"("Desired Angle"=0.0, "Encoder Distance (in.)"=10.0 ("Encoder Distance")) -> ("Stop"=w313:bool)  [unwired: 9 in]
                              }
                              n359 = while {
                                stop <- w311 stop-if-true
                                n360 = call "Auto Arms Down V.3.0.vi"() -> ("Stop"=w311:bool)  [unwired: 11 in]
                              }
                            }
                            frame Enabled {
                            }
                          }
                        }
                      }
                    }
                    frame Disabled {
                      n361 = flat-sequence {
                        frame #0 {
                          n362 = call "Reset Encoder V.3.0.vi"() -> ()  [unwired: 12 in]
                        }
                        frame #1 {
                          n363 = while {
                            stop <- w316 stop-if-true
                            # "Forward"
                            n364 = call "Drive Backward V.3.0.vi"("Desired Angle"=0.0, "Encoder Distance (in.)"=-232) -> ("Stop"=w316:bool)  [unwired: 9 in]
                          }
                        }
                        frame #2 {
                          n365 = while {
                            stop <- w319 stop-if-true
                            # "Right"
                            n366 = call "Right Auto V.3.0.vi"("Desired Angle"=90) -> ("Stop"=w319:bool)  [unwired: 9 in]
                          }
                        }
                        frame #3 {
                          n367 = call "Reset Encoder V.3.0.vi"() -> ()  [unwired: 12 in]
                        }
                        frame #4 {
                          n368 = while {
                            stop <- w321 stop-if-true
                            # "Forward"
                            n369 = call "Drive Backward V.3.0.vi"("Desired Angle"=90.0, "Encoder Distance (in.)"=-200) -> ("Stop"=w321:bool)  [unwired: 9 in]
                          }
                        }
                        frame #5 {
                          n370 = flat-sequence {
                            frame #0 {
                              n371 = while {
                                stop <- w325 stop-if-true
                                # "Left"
                                n372 = call "Left Auto V.3.0.vi"("Desired Angle"=0) -> ("Stop"=w325:bool)  [unwired: 10 in]
                              }
                            }
                            frame #1 {
                              n373 = call "Reset Encoder V.3.0.vi"() -> ()  [unwired: 12 in]
                            }
                            frame #2 {
                              n374 = while {
                                stop <- w328 stop-if-true
                                # "Forward"
                                n375 = call "Drive Backward V.3.0.vi"("Desired Angle"=0.0, "Encoder Distance (in.)"=-49) -> ("Stop"=w328:bool)  [unwired: 9 in]
                              }
                            }
                          }
                          n376 = while {
                            stop <- w323 stop-if-true
                            # "Raise Darts"
                            n377 = call "Dart Auto V.3.0.vi"() -> ("Stop"=w323:bool)  [unwired: 11 in]
                          }
                        }
                      }
                    }
                  }
                }
              }
            }
            frame "Nothing", Default {
            }
          }
        }
        frame "Right Start Always Scale" {
          w329 = 1 ("length (rest)")
          n378 = call <vilib>:"WPI_DriverStationGame Specific Data.vi"() -> ("Game Specific Data"=w331:string)  [unwired: 11 in]
          n379 = String Subset(string=w331, offset (0)=w329, length (rest)=w329) -> (substring=w330:string)
          n380 = case shown="\"R\"" w330 {
            frame "L" {
              n381 = flat-sequence {
                frame #0 {
                  n382 = call "Reset Encoder V.3.0.vi"() -> ()  [unwired: 12 in]
                }
                frame #1 {
                  n383 = while {
                    stop <- w333 stop-if-true
                    # "Forward"
                    n384 = call "Drive Backward V.3.0.vi"("Desired Angle"=0.0, "Encoder Distance (in.)"=-232) -> ("Stop"=w333:bool)  [unwired: 9 in]
                  }
                }
                frame #2 {
                  n385 = while {
                    stop <- w336 stop-if-true
                    # "Right"
                    n386 = call "Left Auto V.3.0.vi"("Desired Angle"=-90) -> ("Stop"=w336:bool)  [unwired: 10 in]
                  }
                }
                frame #3 {
                  n387 = call "Reset Encoder V.3.0.vi"() -> ()  [unwired: 12 in]
                }
                frame #4 {
                  n388 = while {
                    stop <- w338 stop-if-true
                    # "Forward"
                    n389 = call "Drive Backward V.3.0.vi"("Desired Angle"=-90.0, "Encoder Distance (in.)"=-200) -> ("Stop"=w338:bool)  [unwired: 9 in]
                  }
                }
                frame #5 {
                  n390 = flat-sequence {
                    frame #0 {
                      n391 = while {
                        stop <- w342 stop-if-true
                        # "Left"
                        n392 = call "Right Auto V.3.0.vi"("Desired Angle"=0) -> ("Stop"=w342:bool)  [unwired: 9 in]
                      }
                    }
                    frame #1 {
                      n393 = call "Reset Encoder V.3.0.vi"() -> ()  [unwired: 12 in]
                    }
                    frame #2 {
                      n394 = disable-structure shown="Disabled" {
                        frame Disabled {
                          n395 = while {
                            stop <- w345 stop-if-true
                            # "Forward"
                            n396 = call "Drive Backward V.3.0.vi"("Desired Angle"=0.0, "Encoder Distance (in.)"=-49) -> ("Stop"=w345:bool)  [unwired: 9 in]
                          }
                        }
                        frame Enabled {
                        }
                      }
                    }
                  }
                  n397 = while {
                    stop <- w340 stop-if-true
                    # "Raise Darts"
                    n398 = call "Dart Auto V.3.0.vi"() -> ("Stop"=w340:bool)  [unwired: 11 in]
                  }
                }
                frame #6 {
                  n399 = disable-structure shown="Disabled" {
                    frame Disabled {
                      n400 = while {
                        i -> [w347]
                        stop <- w346 stop-if-true
                        # "Shoot Cube"
                        n401 = call "Shoot Auto V.3.0.vi"("Iteration"=w347) -> ("Stop"=w346:bool)  [unwired: 10 in]
                      }
                    }
                    frame Enabled {
                    }
                  }
                }
                frame #7 {
                  n402 = call "Reset Encoder V.3.0.vi"() -> ()  [unwired: 12 in]
                }
                frame #8 {
                  n403 = disable-structure shown="Disabled" {
                    frame Disabled {
                      n404 = while {
                        stop <- w350 stop-if-true
                        # "Move Backward"
                        n405 = call "Forward Auto V.3.0.vi"("Desired Angle"=0.0, "Encoder Distance (in.)"=10.0 ("Encoder Distance")) -> ("Stop"=w350:bool)  [unwired: 9 in]
                      }
                      n406 = while {
                        stop <- w348 stop-if-true
                        n407 = call "Auto Arms Down V.3.0.vi"() -> ("Stop"=w348:bool)  [unwired: 11 in]
                      }
                    }
                    frame Enabled {
                    }
                  }
                }
              }
            }
            frame "R" {
              n408 = flat-sequence {
                frame #0 {
                  n409 = call "Reset Encoder V.3.0.vi"() -> ()  [unwired: 12 in]
                }
                frame #1 {
                  # "was -277"
                  n410 = while {
                    stop <- w353 stop-if-true
                    # "You go forward"
                    n411 = call "Drive Backward V.3.0.vi"("Desired Angle"=0.0, "Encoder Distance (in.)"=-262) -> ("Stop"=w353:bool)  [unwired: 9 in]
                  }
                }
                frame #2 {
                  n412 = flat-sequence {
                    frame #0 {
                      n413 = while {
                        stop <- w357 stop-if-true
                        # "Turn LEFT"
                        n414 = call "Left Auto V.3.0.vi"("Desired Angle"=-60) -> ("Stop"=w357:bool)  [unwired: 10 in]
                      }
                    }
                    frame #1 {
                      n415 = call "Reset Encoder V.3.0.vi"() -> ()  [unwired: 12 in]
                    }
                    frame #2 {
                      n416 = while {
                        stop <- w360 stop-if-true
                        # "Forward"
                        n417 = call "Drive Backward V.3.0.vi"("Desired Angle"=-60.0, "Encoder Distance (in.)"=-16) -> ("Stop"=w360:bool)  [unwired: 9 in]
                      }
                    }
                  }
                  n418 = while {
                    stop <- w355 stop-if-true
                    # "Raise Darts"
                    n419 = call "Dart Auto V.3.0.vi"() -> ("Stop"=w355:bool)  [unwired: 11 in]
                  }
                }
                frame #3 {
                  n420 = call "Reset Encoder V.3.0.vi"() -> ()  [unwired: 12 in]
                }
                frame #4 {
                  n421 = disable-structure shown="Enabled" {
                    frame Enabled {
                      n422 = while {
                        stop <- w365 stop-if-true
                        # "Move Backward"
                        n423 = call "Forward Auto V.3.0.vi"("Desired Angle"=90.0, "Encoder Distance (in.)"=30.0 ("Encoder Distance")) -> ("Stop"=w365:bool)  [unwired: 9 in]
                      }
                      n424 = flat-sequence {
                        frame #0 {
                          n425 = while {
                            i -> [w362]
                            stop <- w361 stop-if-true
                            # "Shoot Cube"
                            n426 = call "Shoot Auto V.3.0.vi"("Iteration"=w362) -> ("Stop"=w361:bool)  [unwired: 10 in]
                          }
                        }
                        frame #1 {
                          n427 = while {
                            stop <- w363 stop-if-true
                            n428 = call "Auto Arms Down V.3.0.vi"() -> ("Stop"=w363:bool)  [unwired: 11 in]
                          }
                        }
                      }
                    }
                    frame Disabled {
                    }
                  }
                }
                frame #5 {
                  n429 = disable-structure shown="Disabled" {
                    frame Disabled {
                      n430 = while {
                        stop <- w368 stop-if-true
                        # "Turn right slightly"
                        n431 = call "Right Auto V.3.0.vi"("Desired Angle"=-30) -> ("Stop"=w368:bool)  [unwired: 9 in]
                      }
                    }
                    frame Enabled {
                    }
                  }
                }
              }
            }
            frame "Nothing", Default {
            }
          }
        }
        frame "Scale Optimize Right Start" {
          w370 = 1 ("length (rest)")
          n432 = call <vilib>:"WPI_DriverStationGame Specific Data.vi"() -> ("Game Specific Data"=w371:string)  [unwired: 11 in]
          n433 = String Subset(string=w371, offset (0)=w370, length (rest)=w370) -> (substring=w369:string)
          n434 = case shown="\"R\"" w369 {
            frame "Nothing", Default {
            }
            frame "L" {
              n435 = call <vilib>:"WPI_DriverStationGame Specific Data.vi"() -> ("Game Specific Data"=w374:string)  [unwired: 11 in]
              n436 = String Subset(string=w374, length (rest)=1 ("length (rest)")) -> (substring=w372:string)  [unwired: 1 in]
              n437 = case shown="\"R\"" w372 {
                frame "Nothing", Default {
                }
                frame "L" {
                  # "both opposite sidez - do scale"
                  n438 = disable-structure shown="Enabled" {
                    frame Enabled {
                      n439 = flat-sequence {
                        frame #0 {
                          n440 = call "Reset Encoder V.3.0.vi"() -> ()  [unwired: 12 in]
                        }
                        frame #1 {
                          n441 = while {
                            stop <- w376 stop-if-true
                            # "Forward"
                            n442 = call "Drive Backward V.3.0.vi"("Desired Angle"=0.0, "Encoder Distance (in.)"=-232) -> ("Stop"=w376:bool)  [unwired: 9 in]
                          }
                        }
                        frame #2 {
                          n443 = while {
                            stop <- w379 stop-if-true
                            # "Right"
                            n444 = call "Left Auto V.3.0.vi"("Desired Angle"=-90) -> ("Stop"=w379:bool)  [unwired: 10 in]
                          }
                        }
                        frame #3 {
                          n445 = call "Reset Encoder V.3.0.vi"() -> ()  [unwired: 12 in]
                        }
                        frame #4 {
                          n446 = while {
                            stop <- w381 stop-if-true
                            # "Forward"
                            n447 = call "Drive Backward V.3.0.vi"("Desired Angle"=-90.0, "Encoder Distance (in.)"=-200) -> ("Stop"=w381:bool)  [unwired: 9 in]
                          }
                        }
                        frame #5 {
                          n448 = flat-sequence {
                            frame #0 {
                              n449 = while {
                                stop <- w385 stop-if-true
                                # "Left"
                                n450 = call "Right Auto V.3.0.vi"("Desired Angle"=0) -> ("Stop"=w385:bool)  [unwired: 9 in]
                              }
                            }
                            frame #1 {
                              n451 = call "Reset Encoder V.3.0.vi"() -> ()  [unwired: 12 in]
                            }
                            frame #2 {
                              n452 = disable-structure shown="Disabled" {
                                frame Disabled {
                                n453 = while {
                                stop <- w388 stop-if-true
                                # "Forward"
                                n454 = call "Drive Backward V.3.0.vi"("Desired Angle"=0.0, "Encoder Distance (in.)"=-49) -> ("Stop"=w388:bool)  [unwired: 9 in]
                                }
                                }
                                frame Enabled {
                                }
                              }
                            }
                          }
                          n455 = while {
                            stop <- w383 stop-if-true
                            # "Raise Darts"
                            n456 = call "Dart Auto V.3.0.vi"() -> ("Stop"=w383:bool)  [unwired: 11 in]
                          }
                        }
                        frame #6 {
                          n457 = disable-structure shown="Disabled" {
                            frame Disabled {
                              n458 = while {
                                i -> [w390]
                                stop <- w389 stop-if-true
                                # "Shoot Cube"
                                n459 = call "Shoot Auto V.3.0.vi"("Iteration"=w390) -> ("Stop"=w389:bool)  [unwired: 10 in]
                              }
                            }
                            frame Enabled {
                            }
                          }
                        }
                        frame #7 {
                          n460 = call "Reset Encoder V.3.0.vi"() -> ()  [unwired: 12 in]
                        }
                        frame #8 {
                          n461 = disable-structure shown="Disabled" {
                            frame Disabled {
                              n462 = while {
                                stop <- w393 stop-if-true
                                # "Move Backward"
                                n463 = call "Forward Auto V.3.0.vi"("Desired Angle"=0.0, "Encoder Distance (in.)"=10.0 ("Encoder Distance")) -> ("Stop"=w393:bool)  [unwired: 9 in]
                              }
                              n464 = while {
                                stop <- w391 stop-if-true
                                n465 = call "Auto Arms Down V.3.0.vi"() -> ("Stop"=w391:bool)  [unwired: 11 in]
                              }
                            }
                            frame Enabled {
                            }
                          }
                        }
                      }
                    }
                    frame Disabled {
                      n466 = flat-sequence {
                        frame #0 {
                          n467 = call "Reset Encoder V.3.0.vi"() -> ()  [unwired: 12 in]
                        }
                        frame #1 {
                          n468 = while {
                            stop <- w396 stop-if-true
                            # "Forward"
                            n469 = call "Drive Backward V.3.0.vi"("Desired Angle"=0.0, "Encoder Distance (in.)"=-232) -> ("Stop"=w396:bool)  [unwired: 9 in]
                          }
                        }
                        frame #2 {
                          n470 = while {
                            stop <- w399 stop-if-true
                            # "Right"
                            n471 = call "Left Auto V.3.0.vi"("Desired Angle"=-90) -> ("Stop"=w399:bool)  [unwired: 10 in]
                          }
                        }
                        frame #3 {
                          n472 = call "Reset Encoder V.3.0.vi"() -> ()  [unwired: 12 in]
                        }
                        frame #4 {
                          n473 = while {
                            stop <- w401 stop-if-true
                            # "Forward"
                            n474 = call "Drive Backward V.3.0.vi"("Desired Angle"=-90.0, "Encoder Distance (in.)"=-200) -> ("Stop"=w401:bool)  [unwired: 9 in]
                          }
                        }
                        frame #5 {
                          n475 = flat-sequence {
                            frame #0 {
                              n476 = while {
                                stop <- w405 stop-if-true
                                # "Left"
                                n477 = call "Right Auto V.3.0.vi"("Desired Angle"=0) -> ("Stop"=w405:bool)  [unwired: 9 in]
                              }
                            }
                            frame #1 {
                              n478 = call "Reset Encoder V.3.0.vi"() -> ()  [unwired: 12 in]
                            }
                            frame #2 {
                              n479 = while {
                                stop <- w408 stop-if-true
                                # "Forward"
                                n480 = call "Drive Backward V.3.0.vi"("Desired Angle"=0.0, "Encoder Distance (in.)"=-49) -> ("Stop"=w408:bool)  [unwired: 9 in]
                              }
                            }
                          }
                          n481 = while {
                            stop <- w403 stop-if-true
                            # "Raise Darts"
                            n482 = call "Dart Auto V.3.0.vi"() -> ("Stop"=w403:bool)  [unwired: 11 in]
                          }
                        }
                      }
                    }
                  }
                }
                frame "R" {
                  # "opposite side scale same side switch - do switch"
                  n483 = flat-sequence {
                    frame #0 {
                      n484 = call "Reset Encoder V.3.0.vi"() -> ()  [unwired: 12 in]
                    }
                    frame #1 {
                      n485 = while {
                        stop <- w411 stop-if-true
                        # "Drive Forward"
                        n486 = call "Drive Backward V.3.0.vi"("Desired Angle"=0.0, "Encoder Distance (in.)"=-162.0) -> ("Stop"=w411:bool)  [unwired: 9 in]
                      }
                    }
                    frame #2 {
                      n487 = while {
                        stop <- w413 stop-if-true
                        # "Turn LEFT"
                        n488 = call "Left Auto V.3.0.vi"("Desired Angle"=-90.0) -> ("Stop"=w413:bool)  [unwired: 10 in]
                      }
                    }
                    frame #3 {
                      n489 = call "Reset Encoder V.3.0.vi"() -> ()  [unwired: 12 in]
                    }
                    frame #4 {
                      n490 = while {
                        stop <- w414 stop-if-true
                        # "Drive Forward"
                        n491 = call "Drive Backward V.3.0.vi"("Desired Angle"=90.0, "Encoder Distance (in.)"=-22.0) -> ("Stop"=w414:bool)  [unwired: 9 in]
                      }
                    }
                    frame #5 {
                      n492 = while {
                        i -> [w417]
                        stop <- w418 stop-if-true
                        # "Shoot"
                        n493 = call "Shoot Auto V.3.0.vi"("Iteration"=w417) -> ("Stop"=w418:bool)  [unwired: 10 in]
                      }
                    }
                  }
                }
              }
            }
            frame "R" {
              # "same side scale, do scale"
              n494 = flat-sequence {
                frame #0 {
                  n495 = call "Reset Encoder V.3.0.vi"() -> ()  [unwired: 12 in]
                }
                frame #1 {
                  # "was -277"
                  n496 = while {
                    stop <- w420 stop-if-true
                    # "You go forward"
                    n497 = call "Drive Backward V.3.0.vi"("Desired Angle"=0.0, "Encoder Distance (in.)"=-262) -> ("Stop"=w420:bool)  [unwired: 9 in]
                  }
                }
                frame #2 {
                  n498 = flat-sequence {
                    frame #0 {
                      n499 = while {
                        stop <- w424 stop-if-true
                        # "Turn LEFT"
                        n500 = call "Left Auto V.3.0.vi"("Desired Angle"=-60) -> ("Stop"=w424:bool)  [unwired: 10 in]
                      }
                    }
                    frame #1 {
                      n501 = call "Reset Encoder V.3.0.vi"() -> ()  [unwired: 12 in]
                    }
                    frame #2 {
                      n502 = while {
                        stop <- w427 stop-if-true
                        # "Forward"
                        n503 = call "Drive Backward V.3.0.vi"("Desired Angle"=-60.0, "Encoder Distance (in.)"=-16) -> ("Stop"=w427:bool)  [unwired: 9 in]
                      }
                    }
                  }
                  n504 = while {
                    stop <- w422 stop-if-true
                    # "Raise Darts"
                    n505 = call "Dart Auto V.3.0.vi"() -> ("Stop"=w422:bool)  [unwired: 11 in]
                  }
                }
                frame #3 {
                  n506 = call "Reset Encoder V.3.0.vi"() -> ()  [unwired: 12 in]
                }
                frame #4 {
                  n507 = disable-structure shown="Enabled" {
                    frame Enabled {
                      n508 = while {
                        stop <- w432 stop-if-true
                        # "Move Backward"
                        n509 = call "Forward Auto V.3.0.vi"("Desired Angle"=90.0, "Encoder Distance (in.)"=30.0 ("Encoder Distance")) -> ("Stop"=w432:bool)  [unwired: 9 in]
                      }
                      n510 = flat-sequence {
                        frame #0 {
                          n511 = while {
                            i -> [w429]
                            stop <- w428 stop-if-true
                            # "Shoot Cube"
                            n512 = call "Shoot Auto V.3.0.vi"("Iteration"=w429) -> ("Stop"=w428:bool)  [unwired: 10 in]
                          }
                        }
                        frame #1 {
                          n513 = while {
                            stop <- w430 stop-if-true
                            n514 = call "Auto Arms Down V.3.0.vi"() -> ("Stop"=w430:bool)  [unwired: 11 in]
                          }
                        }
                      }
                    }
                    frame Disabled {
                    }
                  }
                }
                frame #5 {
                  n515 = disable-structure shown="Disabled" {
                    frame Disabled {
                      n516 = while {
                        stop <- w435 stop-if-true
                        # "Turn right slightly"
                        n517 = call "Right Auto V.3.0.vi"("Desired Angle"=-30) -> ("Stop"=w435:bool)  [unwired: 9 in]
                      }
                    }
                    frame Enabled {
                    }
                  }
                }
              }
            }
          }
        }
      }
    }
  }
  n518 = while {
    stop <- FALSE stop-if-true
    n519 = call <vilib>:"WPI_DriverStationReport Robot Code State.vi"("Autonomous"=TRUE) -> ()  [unwired: 10 in, 1 out]
    n520 = Wait (ms)(milliseconds to wait=u32 20) -> ()  [unwired: 1 out]
  }
